vi "Task Stop.vi"(8 "error in (no error)":errorcluster, 11 "DebugGUI in":refnum<class "DebugGUI.lvclass">) -> (0 "error out":errorcluster, 3 "DebugGUI out":refnum<class "DebugGUI.lvclass">)   [LabVIEW 2020, in "Volatus.lvlib" / "DebugGUI.lvclass"]
uses:
  DebugGUI.lvclass
  DebugGUI.lvclass/DebugGUI.ctl
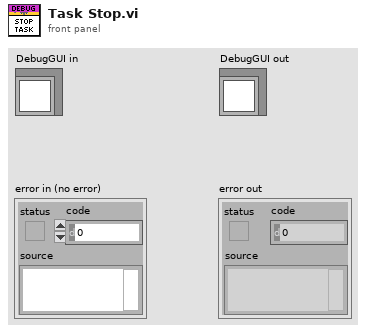
[diagram p1: front panel]
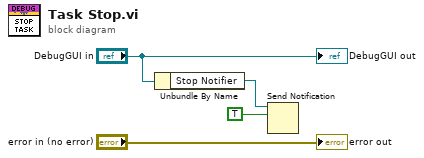
[diagram p0: block diagram]
diagram:
  n1 = Unbundle By Name("DebugGUI in") -> ("Stop Notifier"=w2:refnum<notifier>)
  n2 = Send Notification(notification=TRUE, notifier=w2) -> ()  [unwired: 1 in, 2 out]
  "error out" <- "error in (no error)"
  "DebugGUI out" <- "DebugGUI in"
